vi "C13HLAverager.vi"(9 "Block Data":T1, 10 "low limit":dbl, 11 "CurPoints":i32) -> (1 "13CCurrent":bool, 2 "C13HL":dbl)   [LabVIEW 2013]
uses:
  ctl/BlockData.ctl
  <vilib>/Analysis/baseanly.llb/Mean (DBL).vi
  <vilib>/Analysis/NI_AALBase.lvlib
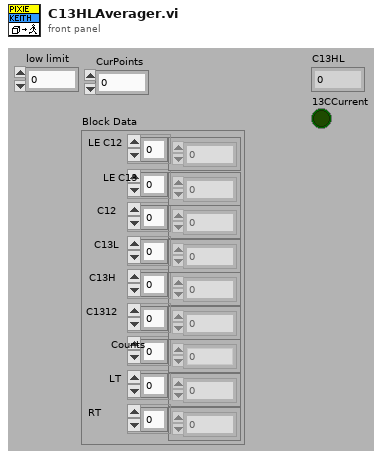
[diagram p1: front panel]
types:
  T1 = typedef "BlockData.ctl" = cluster{"LE C12":dbl[], "LE C13":dbl[], "C12":dbl[], "C13L":dbl[], "C13H":dbl[], "C1312":dbl[], "Counts":u32[], "LT":dbl[], "RT":dbl[]}
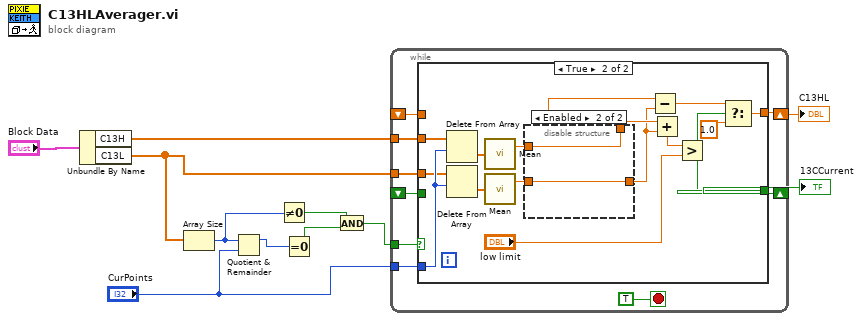
[diagram p0: block diagram]
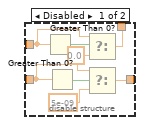
[diagram p3: hidden frame]
diagram:
  n1 = Unbundle By Name("Block Data") -> ("C13H"=w10:dbl[], "C13L"=w8:dbl[])
  n2 = Array Size(array=w8) -> (size(s)=w5:i32)
  n3 = Quotient & Remainder(x=w5, y="CurPoints") -> (x-y*floor(x/y)=w2:i32)  [unwired: 1 out]
  n4 = Not Equal To 0?(x=w5) -> (x != 0?=w6:bool)
  n5 = Equal To 0?(x=w2) -> (x = 0?=w3:bool)
  n6 = And(x=w6, y=w3) -> (x .and. y?=w4:bool)
  n7 = while {
    tunnel: "CurPoints" -> [w20]
    tunnel: w8 -> [w19]
    tunnel: w10 -> [w18]
    tunnel: w4 -> [w17]
    shift-right: [w16] -> w9
    shift-left: _ -> [w14]
    shift-right: [w13] -> w1
    shift-left: _ -> [w12]
    stop <- TRUE stop-if-true
    n8 = case shown="True" w17 {
      tunnel: w20 -> [_ w35]
      tunnel: w18 -> [_ w34]
      tunnel: w19 -> [_ w33]
      tunnel: [w22 w31] -> w16
      tunnel: w14 -> [w22 _]
      tunnel: [w21 w28] -> w13
      tunnel: w12 -> [w21 _]
      frame False {
      }
      frame True {
        n9 = Delete From Array(array=w34, length=w35) -> (deleted portion=w37:dbl[])  [unwired: 1 in, 1 out]
        n10 = Delete From Array(array=w33, length=w35) -> (deleted portion=w36:dbl[])  [unwired: 1 in, 1 out]
        n11 = call-poly <vilib>:"Mean.vi"("X"=w37) -> ("mean"=w23:dbl)  [unwired: 1 out]
        n12 = call-poly <vilib>:"Mean.vi"("X"=w36) -> ("mean"=w24:dbl)  [unwired: 1 out]
        n13 = disable-structure shown="Enabled" {
          disable-tunnel: [w44 w47] -> w26
          disable-tunnel: [w43 w46] -> w25
          disable-tunnel: w24 -> [w41 w46]
          disable-tunnel: w23 -> [w40 w47]
          frame Disabled {
            n14 = Greater Than 0?(x=w40) -> (x > 0?=w45:bool)
            n15 = Greater Than 0?(x=w41) -> (x > 0?=w42:bool)
            n16 = Select(t=w40, s=w45, f=0.0) -> (s? t:f=w44:dbl)
            n17 = Select(t=w41, s=w42, f=5e-09) -> (s? t:f=w43:dbl)
          }
          frame Enabled {
          }
        }
        n18 = Subtract(x=w26, y=w25) -> (x-y=w32:dbl)
        n19 = Add(x=w26, y=w25) -> (x+y=w27:dbl)
        n20 = Greater?(x=w27, y="low limit") -> (0:w28:bool)
        n21 = Select(t=w32, s=w28, f=1.0) -> (s? t:f=w31:dbl)
      }
    }
  }
  "C13HL" <- w9
  "13CCurrent" <- w1
